vi "Fill Maps.vi"(5 "User Events":T1, 7 "Project Selected":string="DQMH Modules", 10 "Module names":string[](array[string]), 11 "DQMH Modules":refnum<vi>[](array[refnum])) -> (1 "Cancelled?":bool, 2 "map ref out":map{string, refnum<vi>}(c390), 3 "Tree Map out":T2)   [LabVIEW 2020, in "Dashboard.lvlib"]
uses:
  Dashboard.lvlib
  <vilib>/National Instruments/Tree Map/Tree Map Data.ctl
  Panther Dashboard Project/support/User Event - Stop/User Events Refs--cluster.ctl
  Event types--enum.ctl
  <vilib>/National Instruments/Tree Map/Tree Map.lvlib
  Panther Dashboard Project/support/User Event - Stop/User Events.lvlib
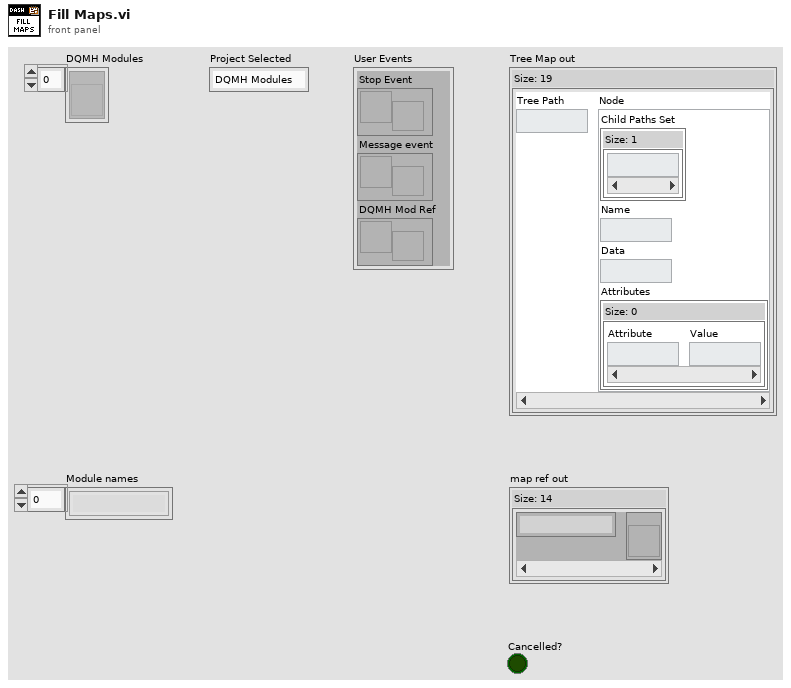
[diagram p1: front panel]
types:
  T1 = typedef "User Events.lvlib/User Events Refs--cluster.ctl" = cluster{"Stop Event":refnum<user-event>, "Message event ":refnum<user-event>, "DQMH Mod Ref":refnum<user-event>}
  T2 = typedef "Tree Map.lvlib/Tree Map Data.ctl" = map{string, cluster{"Child Paths Set":set{string}, "Name":string, "Data":string, "Attributes":map{string, string}}}
  T3 = typedef "Dashboard.lvlib/Event types--enum.ctl" = enum16{"Request", "Request and Wait for Reply", "Broadcast"}
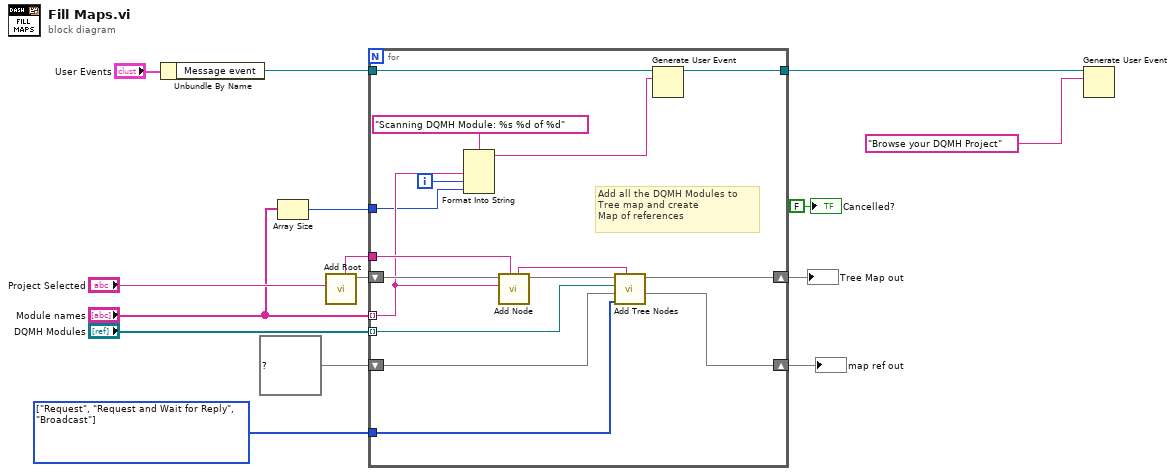
[diagram p0: block diagram]
diagram:
  w8 = T3[] [enum."Request", enum."Request and Wait for Reply", enum."Broadcast"] items=["Request", "Request and Wait for Reply", "Broadcast"] ("Event Types")
  n1 = Unbundle By Name("User Events") -> ("Message event"=w4:refnum<user-event>)
  n2 = Array Size(array="Module names") -> (size(s)=w1:i32)
  n3 = call <vilib>:"Add Root.vi"("New Root Name"="Project Selected") -> ("Tree Map Out"=w11:T2, "Root Path"=w9:string)  [unwired: 9 in]
  n4 = for {
    shift-right: [w29] -> w12
    shift-left: w11 -> [w27]
    shift-right: [w31] -> w14
    shift-left: map{string, refnum<vi>} {} ("References Map") -> [w30]
    tunnel: "DQMH Modules" -> [w23] mode=indexing
    tunnel: w9 -> [w25]
    tunnel: w8 -> [w28]
    tunnel: "Module names" -> [w20] mode=indexing
    tunnel: w4 -> [w22]
    tunnel: [w21] -> w3
    tunnel: w1 -> [w18]
    i -> [w19]
    # "Add all the DQMH Modules to\nTree map and create \nMap of references"
    n5 = Format Into String(format string="Scanning DQMH Module: %s %d of %d", w20, w19, w18) -> (resulting string=w16:string)  [unwired: 2 in, 1 out]
    n6 = call <vilib>:"Add Node.vi"("Parent Path"=w25, "New Node Name"=w20, "Tree Map In"=w27) -> ("Tree Map Out"=w26:T2, "New Node Path"=w24:string)  [unwired: 6 in, 1 out]
    n7 = call "Add Tree Nodes.vi"("Root path"=w24, "Event Types"=w28, "map ref in"=w30, "DQMH Lib In"=w23, "Tree Map in"=w26) -> ("map ref out"=w31:map{string, refnum<vi>}, "Tree Map out"=w29:T2)  [unwired: 5 in]
    n8 = Generate User Event(user event=w22, event data cluster=w16) -> (user event out=w21:refnum<user-event>)  [unwired: 2 in, 1 out]
  }
  "map ref out" <- w14
  "Tree Map out" <- w12
  n9 = Generate User Event(user event=w3, event data cluster="Browse your DQMH Project" ("format string")) -> ()  [unwired: 2 in, 2 out]
  "Cancelled?" <- FALSE ("Cancelled?")
